vi "Plot_Command_File.vi"() -> ()   [LabVIEW 2010]
uses:
  Trav_mode.ctl
  Controls/Multi_run_mode.ctl
  Globals/Trav_pos_global.vi
panel:
  out "No of rows":i32
  in  "Speed Factor":dbl=1.0 min=0.1 max=5.0 format="%.2f"
  in  "Coordinate rotation (deg)":dbl format="%.2f"
  in  "Command filename":path
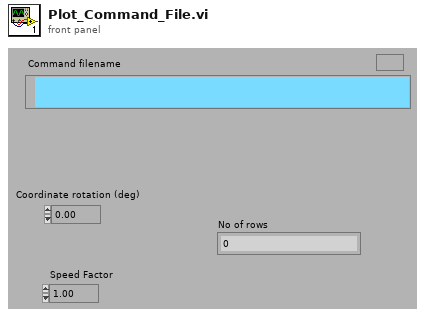
[diagram p1: front panel]
types:
  T1 = typedef "Trav_mode.ctl" = enum16{"Move traverse", "Read traverse position", "Teach Position"}
  T2 = typedef "Multi_run_mode.ctl" = enum16{"Move Traverse Only", "Set Tunnel Speed Only", "Set Source Only", "Set Measurement Conditions", "Single Measurement", "Vertical Profile", "Lateral Profile", "Longitudinal Profile", "Explore Volume", "Multi-Axis Profile", "Auto Calibrate", "Meas Fast FID Bkgnd", "Check Beam Power", "Scanning Valve Measurement", "Run VI Named:", "Set ADAM Ch", "Wait (minutes)", "Send Message", "Synchronize With:", "Fall Back to this Row", "Turn Off Row Repeating", "Blank Row"}
  T3 = typedef "Traverse_cluster.ctl" = cluster{"Start X":dbl, "Start Y":dbl, "Start Z":dbl, "End X":dbl, "End Y":dbl, "End Z":dbl, "No. of pts.":i32, "Spacing":T4, "Filename":path, "Tunnel Speed":dbl, "Averaging time (min)":dbl, "Extra Commands":string, "Specific Arguments":string, "Emission Rate (l/min)":dbl, "Trace Gas Concentration (%)":dbl, "Density Ratio":string, "Comments":string, "Row No":i32, "Row Type Selector":T2, "Completion time":string, "Row Duration (mins)":dbl, "No. of Valid pts.":i32, "Meas Setup File":string}
  T4 = typedef "Spacing.ctl" = enum16{"Linear", "Log", "Gauss", "Specified", "N/A"}
  T5 = typedef "Tunnel_Coordinates.ctl" = enum16{"Work in Tunnel Coordinates", "Work in Model Coordinates"}
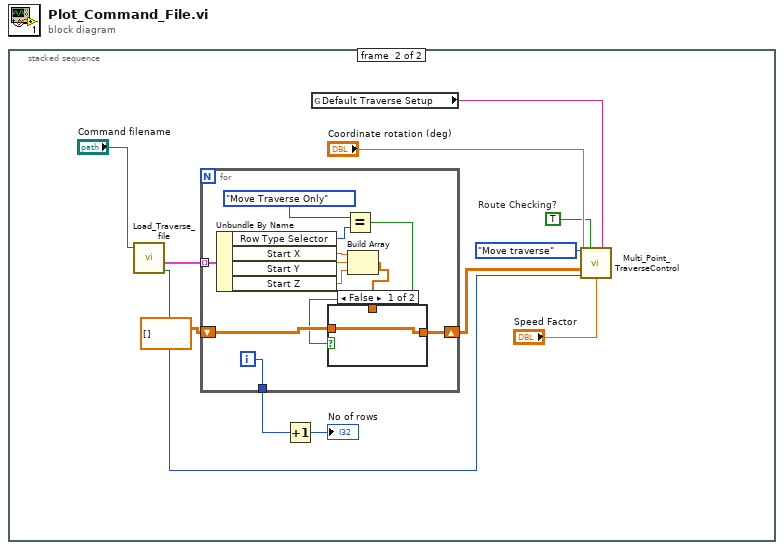
[diagram p0: block diagram]
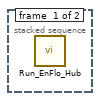
[diagram p2: hidden frame]
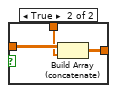
[diagram p3: hidden frame]
diagram:
  n1 = stacked-sequence {
    frame #0 {
      n2 = call "Run_EnFlo_Hub.vi"() -> ()  [unwired: 8 out]
    }
    frame #1 {
      w8 = TRUE  # Route Checking?
      n3 = call "Load_Traverse_file.vi"("Setup filename"="Command filename") -> ("Table"=w11:T3[], "Work in Tunnel Coordinates?"=w6:T5)  [unwired: 4 out]
      n4 = for {
        tunnel: w11 -> [w23] mode=indexing
        tunnel: [w19] -> w5
        shift-right: [w14] -> w1
        shift-left: dbl[][] [] -> [w16]
        i -> [w19]
        n5 = Unbundle By Name(w23) -> ("Row Type Selector"=w17:T2, "Start X"=w21:dbl, "Start Y"=w22:dbl, "Start Z"=w20:dbl)
        n6 = Equal?(x=Multi_run_mode."Move Traverse Only" ("Row Type Selector"), y=w17) -> (x = y?=w13:bool)
        n7 = Build Array(w21, w22, w20) -> (w15:dbl[])
        n8 = case shown="False" w13 {
          tunnel: w16 -> [w24 w27]
          tunnel: w15 -> [_ w26]
          tunnel: [w24 w25] -> w14
          frame False {
          }
          frame True {
            n9 = Build Array (concatenate)(w27, w26) -> (w25:dbl[][])
          }
        }
      }
      n10 = Increment(x=w5) -> (x+1=→"No of rows":i32)
      n11 = global read "Trav_pos_global.vi" "Default Traverse Setup"() -> (w7:string)
      n12 = call "Multi_Point_TraverseControl.vi"("Mode"=Trav_mode."Move traverse", "Route Checking?"=w8, "Traverse Name"=w7, "Coordinate rotation (deg)"="Coordinate rotation (deg)", "Points to plot"=w1, "Work in Tunnel Coordinates?"=w6, "Speed Factor"="Speed Factor") -> ()  [unwired: 1 in, 8 out]
    }
  }
